vi "Results.vi"(8 "error in (no error)":errorcluster, 11 "PmuAnalysis in":refnum<class "PmuAnalysis.lvclass">) -> (0 "error out":errorcluster, 3 "PmuAnalysis out":refnum<class "PmuAnalysis.lvclass">)   [LabVIEW 2014, in "AnalysisPlugins.lvlib" / "PmuAnalysis.lvclass"]
uses:
  PmuAnalysis.lvclass
  AnalysisPluginBaseClass/AnalysisPluginsBase.lvclass
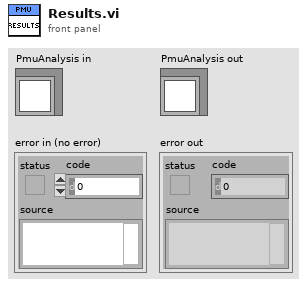
[diagram p1: front panel]
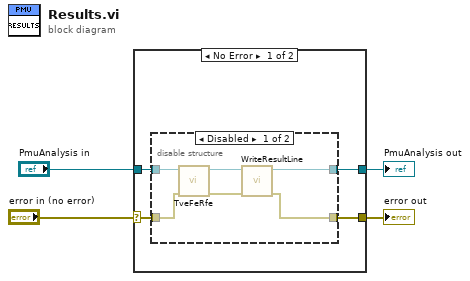
[diagram p0: block diagram]
diagram:
  n1 = case shown="No Error" "error in (no error)" {
    selector: "error in (no error)" -> [w7 w17]
    tunnel: [w6 w18] -> w2
    tunnel: "PmuAnalysis in" -> [w8 w18]
    tunnel: [w5 w17] -> w1
    frame No Error {
      n2 = disable-structure shown="Disabled" {
        disable-tunnel: w8 -> [w14 w16]
        disable-tunnel: w7 -> [w13 w15]
        disable-tunnel: [w11 w16] -> w6
        disable-tunnel: [w9 w15] -> w5
        frame Disabled {
          n3 = call "TveFeRfe.vi"("error in (no error)"=w13, "PmuAnalysis in"=w14) -> ("error out"=w10:errorcluster, "PmuAnalysis out"=w12:refnum<class "PmuAnalysis.lvclass">)  [unwired: 8 in]
          n4 = call "WriteResultLine.vi"("error in (no error)"=w10, "AnalysisPluginsBase in"=w12) -> ("error out"=w9:errorcluster, "AnalysisPluginsBase out"=w11:refnum<class "PmuAnalysis.lvclass">)  [unwired: 8 in]
        }
        frame Enabled {
        }
      }
    }
    frame Error {
    }
  }
  "error out" <- w1
  "PmuAnalysis out" <- w2
